vi "PAN_DBS_precision.vi"(10 "args in":string) -> (1 "precision":i32, 2 "args out":string)   [LabVIEW 2016]
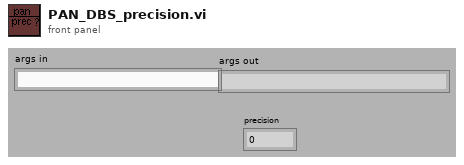
[diagram p1: front panel]
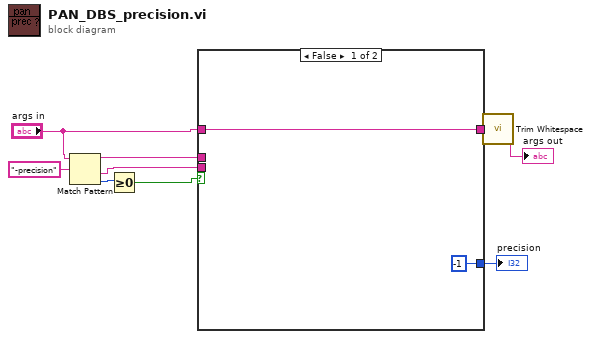
[diagram p0: block diagram]
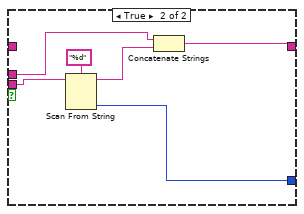
[diagram p2: hidden frame]
diagram:
  n1 = Match Pattern(string="args in", regular expression="-precision") -> (before substring=w6:string, after substring=w5:string, offset past match=w8:i32)  [unwired: 2 out]
  n2 = Greater Or Equal To 0?(x=w8) -> (x >= 0?=w2:bool)
  n3 = case shown="False" w2 {
    tunnel: "args in" -> [w11 _]
    tunnel: [w11 w12] -> w7
    tunnel: w6 -> [_ w14]
    tunnel: w5 -> [_ w17]
    tunnel: [-1 w15] -> w1
    frame False {
    }
    frame True {
      n4 = Scan From String(format string="%d", input string=w17) -> (remaining string=w13:string, output 1=w15:i32)  [unwired: 2 in, 3 out]
      n5 = Concatenate Strings(w14, w13) -> (w12:string)
    }
  }
  "precision" <- w1
  n6 = call <vilib>:"Trim Whitespace.vi"("string"=w7) -> ("trimmed string"=→"args out":string)  [unwired: 1 in]
